vi "Read_XML-File_001.vi"() -> ()   [LabVIEW 2017]
uses:
  D:/MS Project/MS Project/bin/Debug/Ballard_BTI_XML_Deserializer.dll
  MS Project/bin/Debug/Ballard_BTI_XML_Deserializer.dll
panel:
  in  "XML Schema File Path":path=path "\\\\Vboxsvr\\2017/XML Files/BTI.XSD"
  in  "XML Configuration File Path":path=path "\\\\Vboxsvr\\2017/XML Files/XML_000.XML"
  in  "error in (no error)":errorcluster
  out "Array 9":i32[](array[numeric])
  out "Array 8":i32[](array[numeric])
  out "Array 7":string[](array[string])
  out "Array 6":i32[](array[numeric])
  out "Array 5":string[](array[string])
  out "rawData":u8[][](array[numeric])
  out "Array 4":string[](array[string])
  out "Array 2":i32[](array[numeric])
  out "Array":string[](array[string])
  out "error out":errorcluster
  out "name":string
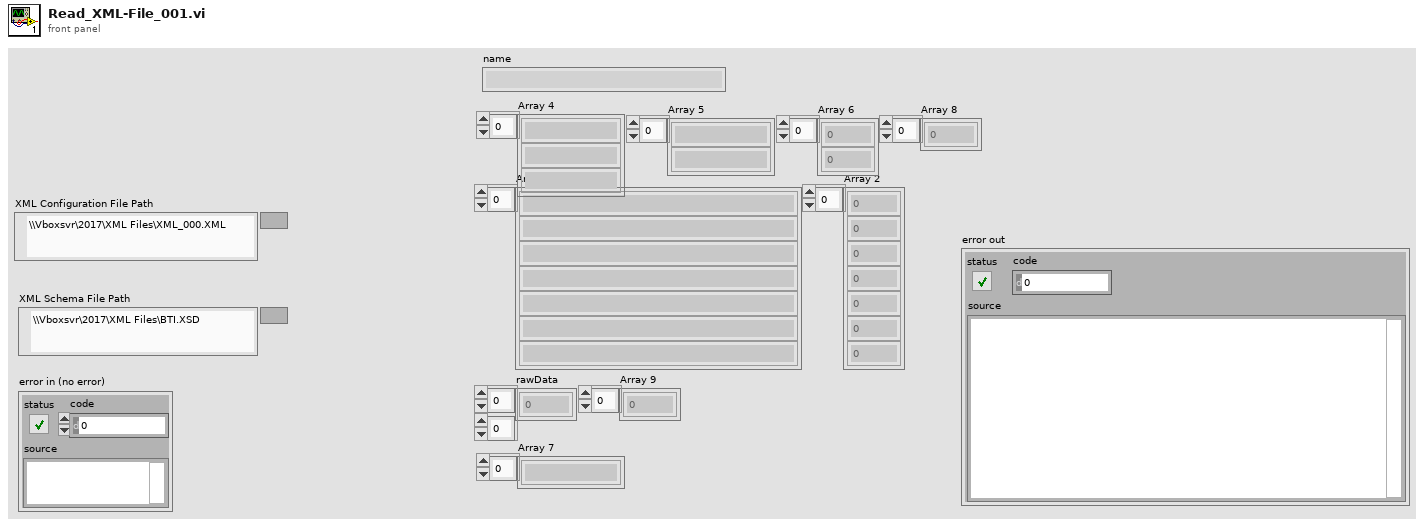
[diagram p1: front panel]
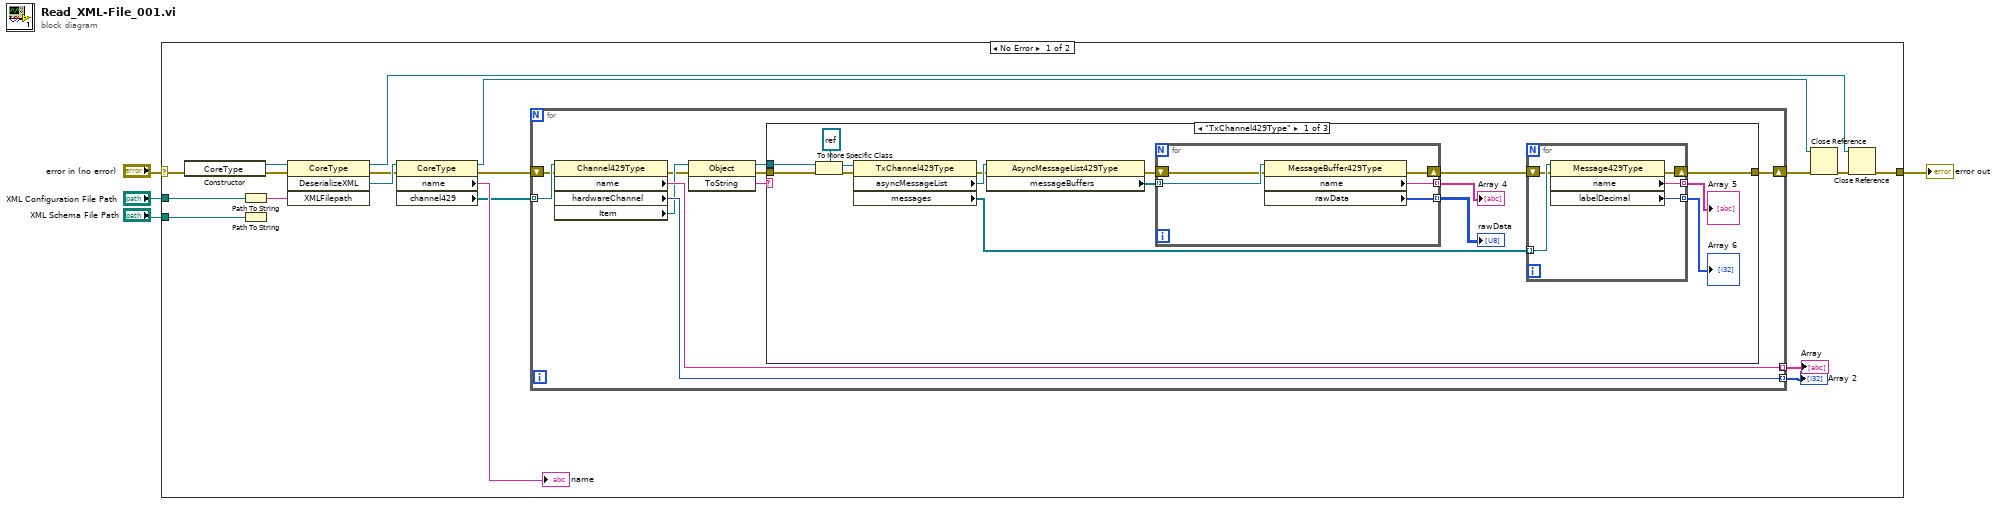
[diagram p0: block diagram]
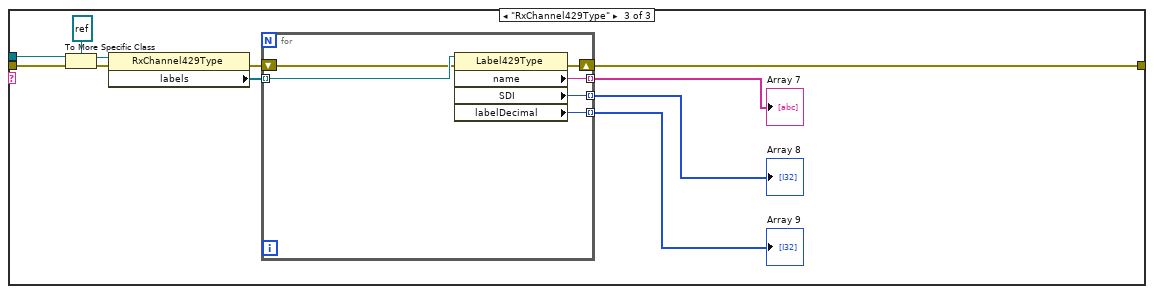
[diagram p3: hidden frame]
diagram:
  n1 = case shown="No Error" "error in (no error)" {
    selector: "error in (no error)" -> [w5 w77]
    tunnel: "XML Configuration File Path" -> [w21 _]
    tunnel: "XML Schema File Path" -> [w13 _]
    tunnel: [w7 w77] -> w2
    frame No Error {
      n2 = constructor class="CoreType"(error in=w5) -> (reference out=w12:refnum<k24>, error out=w11:errorcluster)  [unwired: 2 in, 1 out]
      n3 = Path To String(path=w21) -> (string=w22:string)
      n4 = Path To String(path=w13) -> ()  [unwired: 1 out]
      n5 = invoke class="CoreType" method="DeserializeXML"(reference=w12, error in=w11, "XMLFilepath"=w22) -> (reference out=w6:refnum<k24>, error out=w19:errorcluster, "DeserializeXML"=w20:refnum<k24>)  [unwired: 1 in, 1 out]
      n6 = property class="CoreType"(reference=w20, error in=w19) -> (reference out=w9:refnum<k24>, error out=w14:errorcluster, "name"=→"name":string, "channel429"=w17:refnum<k24>[])
      n7 = for {
        tunnel: w17 -> [w30] mode=indexing
        tunnel: [w32] -> w16 mode=indexing
        tunnel: [w31] -> w15 mode=indexing
        shift-right: [w23] -> w10
        shift-left: w14 -> [w26]
        n8 = property class="Channel429Type"(reference=w30, error in=w26) -> (error out=w25:errorcluster, "name"=w32:string, "hardwareChannel"=w31:i32, "Item"=w29:refnum<k24>)  [unwired: 1 out]
        n9 = invoke class="Object" method="ToString"(reference=w29, error in=w25) -> (reference out=w27:refnum<k24>, error out=w24:errorcluster, "ToString"=w28:string)  [unwired: 1 in]
        n10 = case shown="\"TxChannel429Type\"" w28 {
          tunnel: w27 -> [w48 _ w70]
          tunnel: w24 -> [w47 w59 w69]
          tunnel: [w33 w59 w63] -> w23
          frame "TxChannel429Type" {
            n11 = To More Specific Class(target class=refnum<k24> refnum, reference=w48, error in=w47) -> (specific class reference=w44:refnum<k24>, error out=w45:errorcluster)
            n12 = property class="TxChannel429Type"(reference=w44, error in=w45) -> (error out=w42:errorcluster, "asyncMessageList"=w43:refnum<k24>, "messages"=w39:refnum<k24>[])  [unwired: 1 out]
            n13 = property class="AsyncMessageList429Type"(reference=w43, error in=w42) -> (error out=w40:errorcluster, "messageBuffers"=w41:refnum<k24>[])  [unwired: 1 out]
            n14 = for {
              tunnel: w41 -> [w58] mode=indexing
              shift-right: [w56] -> w38
              shift-left: w40 -> [w57]
              tunnel: [w55] -> w37 mode=indexing
              tunnel: [w54] -> w36 mode=indexing
              n15 = property class="MessageBuffer429Type"(reference=w58, error in=w57) -> (error out=w56:errorcluster, "name"=w55:string, "rawData"=w54:u8[])  [unwired: 1 out]
            }
            "Array 4" <- w37
            "rawData" <- w36
            n16 = for {
              tunnel: w39 -> [w53] mode=indexing
              tunnel: [w51] -> w35 mode=indexing
              tunnel: [w50] -> w34 mode=indexing
              shift-right: [w49] -> w33
              shift-left: w38 -> [w52]
              n17 = property class="Message429Type"(reference=w53, error in=w52) -> (error out=w49:errorcluster, "name"=w51:string, "labelDecimal"=w50:i32)  [unwired: 1 out]
            }
            "Array 5" <- w35
            "Array 6" <- w34
          }
          frame "False", Default {
          }
          frame "RxChannel429Type" {
            n18 = To More Specific Class(target class=refnum<k24> refnum, reference=w70, error in=w69) -> (specific class reference=w66:refnum<k24>, error out=w67:errorcluster)
            n19 = property class="RxChannel429Type"(reference=w66, error in=w67) -> (error out=w64:errorcluster, "labels"=w65:refnum<k24>[])  [unwired: 1 out]
            n20 = for {
              tunnel: w65 -> [w76] mode=indexing
              shift-right: [w74] -> w63
              shift-left: w64 -> [w75]
              tunnel: [w73] -> w62 mode=indexing
              tunnel: [w72] -> w61 mode=indexing
              tunnel: [w71] -> w60 mode=indexing
              n21 = property class="Label429Type"(reference=w76, error in=w75) -> (error out=w74:errorcluster, "name"=w73:string, "SDI"=w72:i32, "labelDecimal"=w71:i32)  [unwired: 1 out]
            }
            "Array 7" <- w62
            "Array 8" <- w61
            "Array 9" <- w60
          }
        }
      }
      "Array" <- w16
      "Array 2" <- w15
      n22 = Close Reference(reference=w9, error in (no error)=w10) -> (error out=w8:errorcluster)
      n23 = Close Reference(reference=w6, error in (no error)=w8) -> (error out=w7:errorcluster)
    }
    frame Error {
    }
  }
  "error out" <- w2
